vi "InsertData.vi"(8 "error in (no error)":errorcluster, 10 "Data Cluster":variant, 11 "object in":refnum<class "TableLogger_SQLite_Actor.lvclass">) -> (0 "error out":errorcluster, 3 "object out":refnum<class "TableLogger_SQLite_Actor.lvclass">)   [LabVIEW 2015, in "TableLogger_SQLite_Actor.lvlib" / "TableLogger_SQLite_Actor.lvclass"]
uses:
  TableLogger_SQLite_Actor.lvclass
  TableLogger_SQLite_Actor.lvclass/TableLogger_SQLite_Actor.ctl
  <vilib>/drjdpowell/SQLite Library/SQL Connection/Execute SQL (No results).vi
  TableLogger_Actor/TableLogger_Actor/TableLogger_Actor.lvclass
  <vilib>/drjdpowell/SQLite Library/SQLite.lvlib
  <vilib>/drjdpowell/SQLite Library/SQL Connection/Connection.lvclass
panel:
  # "Connector Pane"
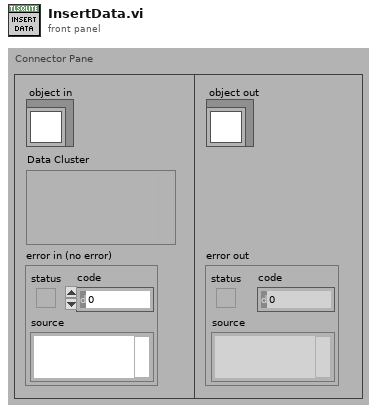
[diagram p1: front panel]
types:
  T1 = typedef "Type Descriptor Enumeration__ogtk.ctl" = enum8{"<Null>", "I8", "I16", "I32", "I64", "U8", "U16", "U32", "U64", "SGL", "DBL", "EXT", "CSG", "CDB", "CXT", "0x0F", "0x10", "0x11", "0x12", "0x13", "0x14", "Enum U8", "Enum U16", "Enum U32", "Enum U64", "SGL PQ", "DBL PQ", "EXT PQ", "CSG PQ", "CDB PQ", "CXT PQ", "0x1F", "0x20", "Boolean", "0x22", "0x23", "0x24", "0x25", "0x26", "0x27", "0x28", "0x29", "0x2A", "0x2B", "0x2C", "0x2D", "0x2E", "0x2F", "String", "0x31", "Path", "Pict", "0x34", "0x35", "0x36", "DAQ", "0x38", "0x39", "0x3A", "0x3B", "0x3C", "0x3D", "0x3E", "0x3F", "Array", "0x41", "0x42", "0x43", "0x44", "0x45", "0x46", "0x47", "0x48", "0x49", "0x4A", "0x4B", "0x4C", "0x4D", "0x4E", "0x4F", "Cluster", "0x51", "0x52", "Variant", "Waveform", "0x55", "0x56", "0x57", "0x58", "0x59", "0x5A", "0x5B", "0x5C", "0x5D", "0x5E", "0x5F", "0x60", "0x61", "0x62", "0x63", "0x64", "0x65", "0x66", "0x67", "0x68", "0x69", "0x6A", "0x6B", "0x6C", "0x6D", "0x6E", "0x6F", "Refnum"}
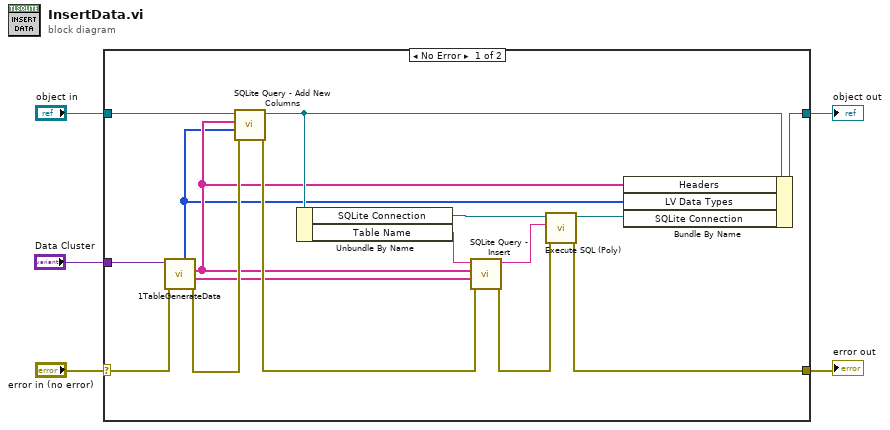
[diagram p0: block diagram]
diagram:
  n1 = case shown="No Error" "error in (no error)" {
    selector: "error in (no error)" -> [w17 w23]
    tunnel: [w14 w23] -> w4
    tunnel: [w19 w22] -> w2
    tunnel: "object in" -> [w20 w22]
    tunnel: "Data Cluster" -> [w18 _]
    frame No Error {
      n2 = call "1TableGenerateData.vi"("error in (no error)"=w17, "Cluster Variant"=w18) -> ("error out"=w16:errorcluster, "Data"=w15:string[], "Headers"=w7:string[], "LV Data Types"=w6:T1[])  [unwired: 5 in, 1 out]
      n3 = call "SQLite Query - Add New Columns.vi"("error in (no error)"=w16, "LV Data Types"=w6, "Headers"=w7, "TableLogger_SQLite_Actor in"=w20) -> ("error out"=w21:errorcluster, "TableLogger_SQLite_Actor out"=w11:refnum<class "TableLogger_SQLite_Actor.lvclass">)  [unwired: 6 in]
      n4 = Unbundle By Name(w11) -> ("SQLite Connection"=w10:refnum<class "Connection.lvclass">, "Table Name"=w8:string)
      n5 = call "SQLite Query - Insert.vi"("error in"=w21, "Data"=w15, "Table Headers"=w7, "Table Name"=w8) -> ("error out"=w9:errorcluster, "SQLite Query"=w12:string)  [unwired: 6 in]
      n6 = call-poly <vilib>:"Execute SQL (Poly).vi"("error in (no error)"=w9, "SQL"=w12, "SQLite Connection in"=w10) -> ("error out"=w14:errorcluster, "SQLite Connection"=w13:refnum<class "Connection.lvclass">)  [unwired: 7 in]
      n7 = Bundle By Name(cluster=w11, "Headers"=w7, "LV Data Types"=w6, "SQLite Connection"=w13) -> (w19:refnum<class "TableLogger_SQLite_Actor.lvclass">)
    }
    frame Error {
    }
  }
  "error out" <- w4
  "object out" <- w2
